vi "ToMotor2CommandSelectFunction.vi"(0 "Switch A Latched":bool=TRUE, 1 "Array":i32[][](array[numeric]), 5 "dt in sec":dbl, 7 "Potentiometer bias (-1 to +1)":dbl, 9 "Encoder 1 count":i64, 11 "Encoder 2 count":i64, 12 "Motor steps 1":i64, 13 "Motor steps 2":i64, 14 "Elapsed Time Out (S)":dbl) -> (4 "Stop":bool, 6 "Motor 1 command":i8=-1, 8 "Motor 2 command":i8=1, 10 "MS lines":bool[](array[boolean]))   [LabVIEW 2014]
panel:
  out "Integer to be added/subtracted":dbl
  out "X0":i32
  out "Y0":i32
  out "X1":i32
  out "Y1":i32
  # "Outputs"
  # "Inputs"
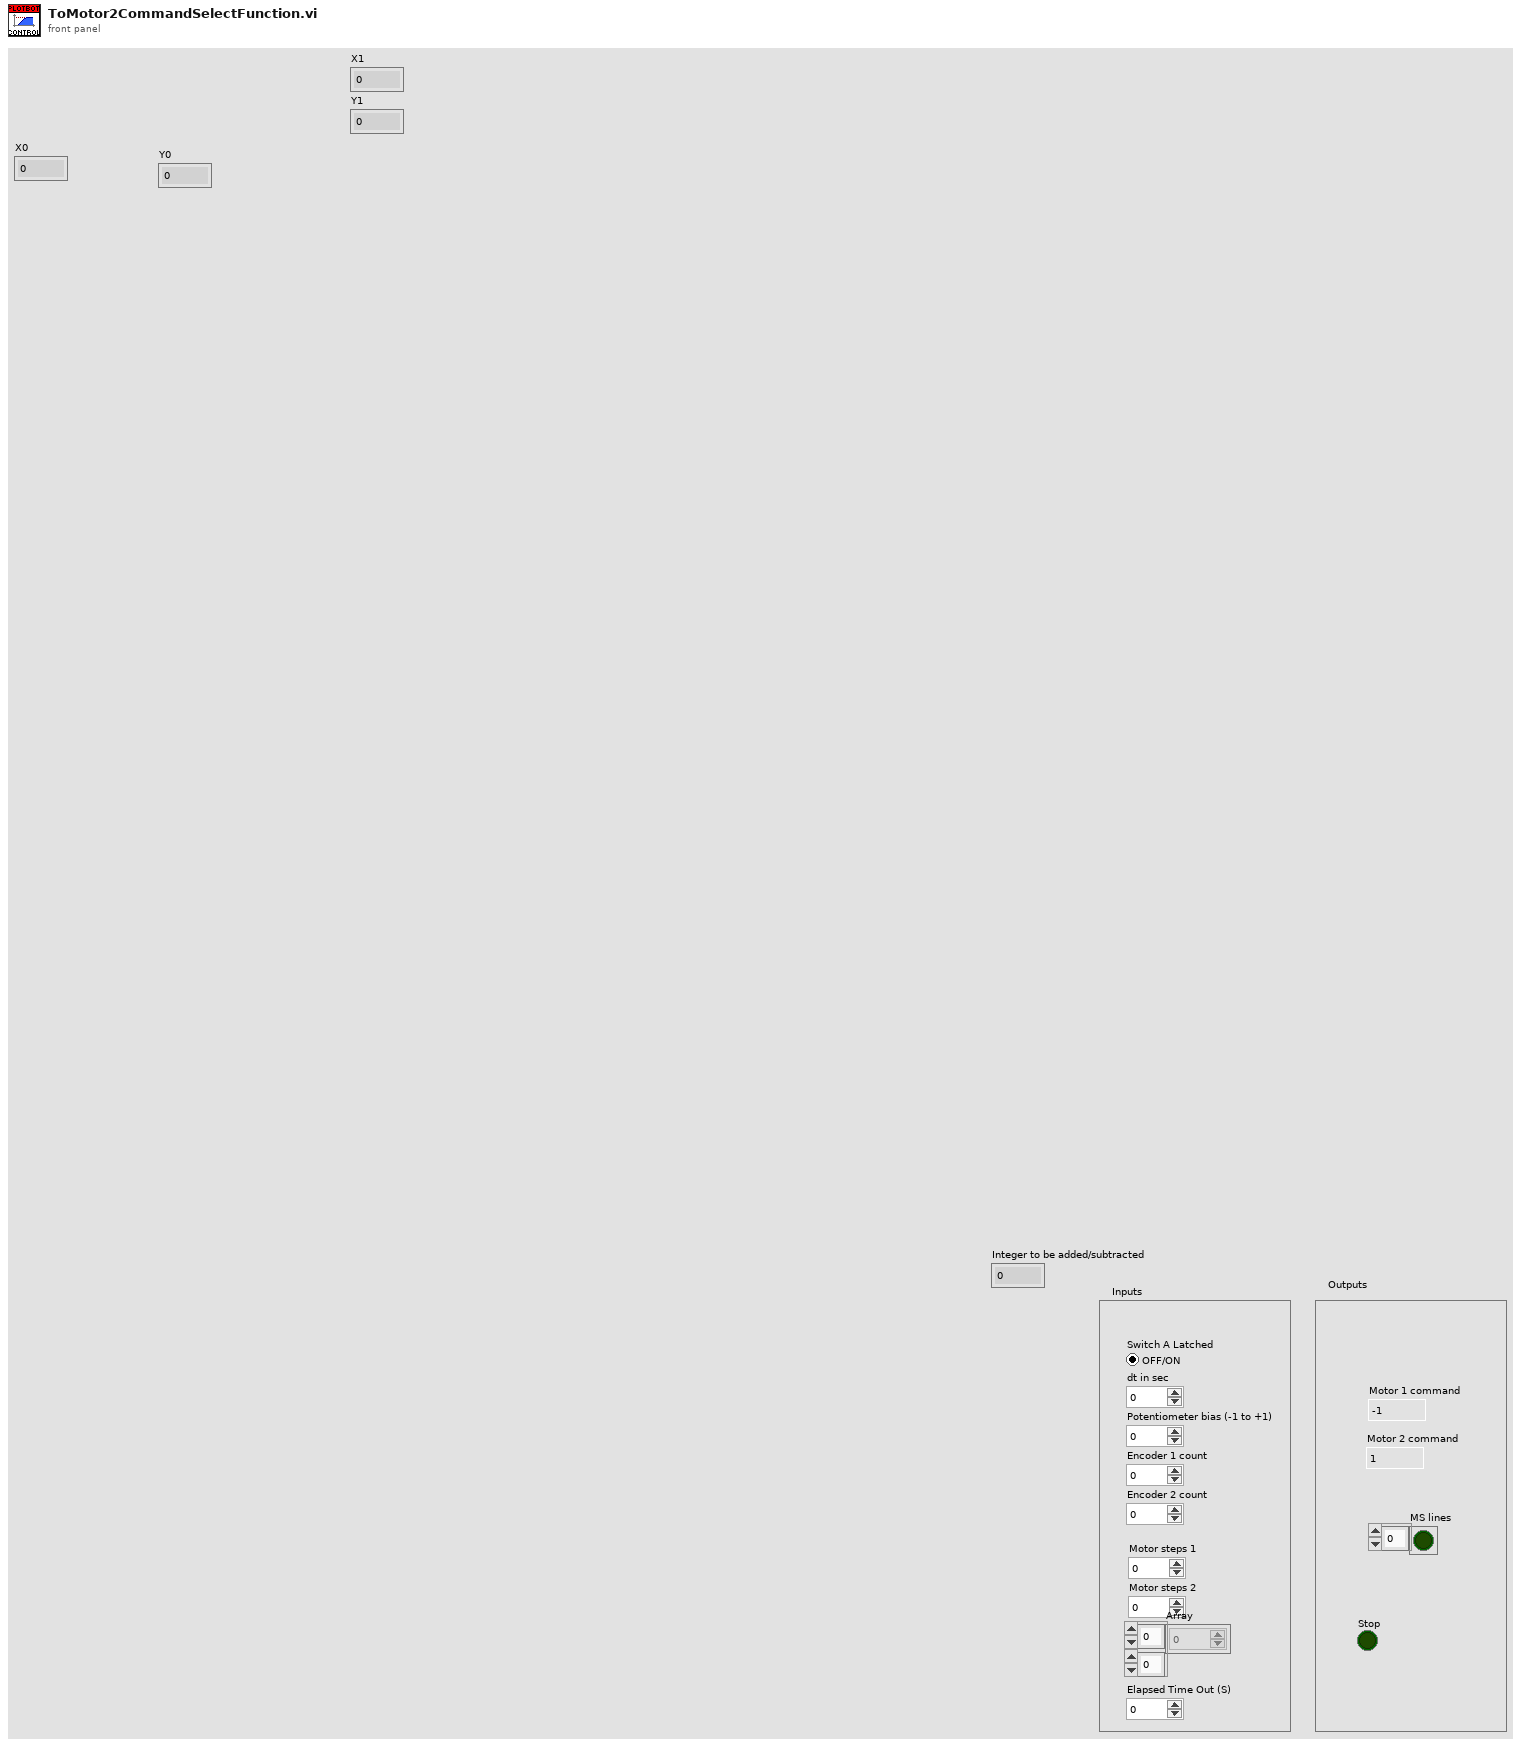
[diagram p1: front panel]
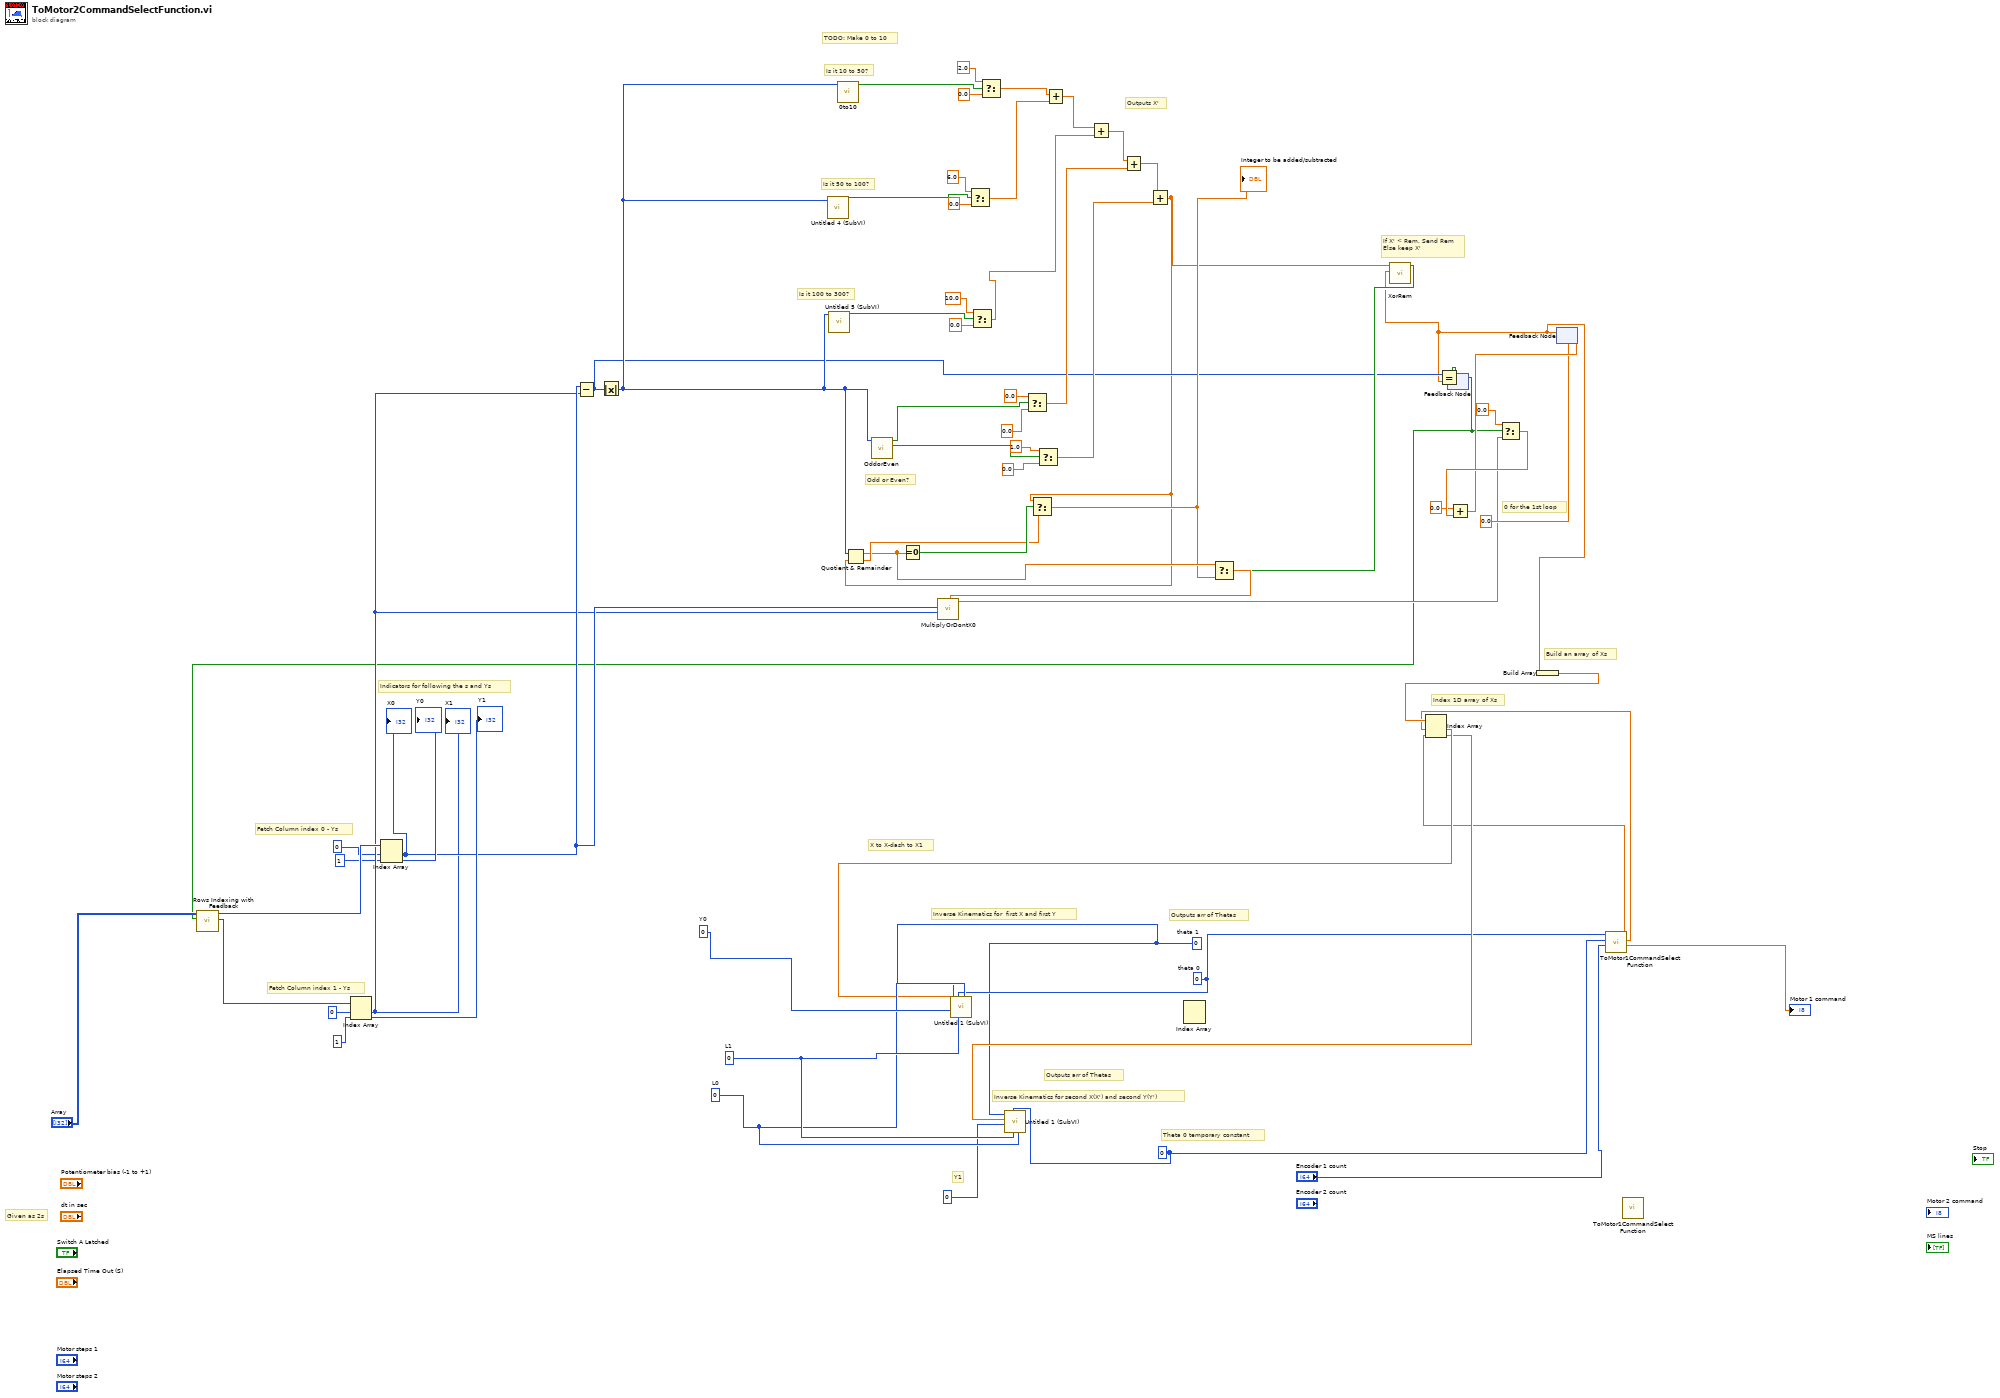
[diagram p0: block diagram]
diagram:
  w5 = 0 ("theta 0")
  w8 = 0  # theta 0
  w6 = 0  # theta 1
  w18 = 0  # L0
  w19 = 0  # L1
  w66 = 0  # Y0
  # "Theta 0 temporary constant"
  # "Y1"
  # "Fetch Column index 1 - Ys"
  # "Fetch Column index 0 - Ys"
  # "Build an array of Xs"
  # "TODO: Make 0 to 10"
  # "Outputs arr of Thetas"
  # "Outputs arr of Thetas"
  # "Inverse Kinematics for second X(X') and second Y(Y')"
  # "X to X-dash to X1"
  # "Inverse Kinematics for  first X and first Y"
  # "Index 1D array of Xs"
  # "Given as 2s"
  # "Outputs X'"
  # "If X' < Rem, Send Rem\nElse keep X'"
  # "Odd or Even?"
  # "Is it 100 to 300?"
  # "Is it 50 to 100?"
  # "Is it 10 to 50?"
  # "0 for the 1st loop"
  # "Indicators for following the s and Ys"
  n1 = Index Array() -> ()  [unwired: 3 in, 2 out]
  n2 = feedback #1() -> (w11:bool)  [unwired: 1 in]
  n3 = call "Rows Indexing with Feedback.vi"("Boolean"=w11, "Array 3"="Array") -> ("Array"=w63:i32[], "Array 2"=w64:i32[])  [unwired: 8 in]
  n4 = Index Array(array=w63, index #1=0 ("index"), index #2=1 ("index")) -> (element #1=w32:i32, element #2=→"Y1":i32)
  "X1" <- w32
  n5 = Index Array(array=w64, index #1=0 ("index"), index #2=1 ("index")) -> (element #1=w33:i32, element #2=→"Y0":i32)
  "X0" <- w33
  n6 = Subtract(x=w33, y=w32) -> (x-y=w23:i32)
  n7 = Absolute Value(x=w23) -> (abs(x)=w30:i32)
  n8 = call "Untitled 4 (SubVI).vi"("Numeric"=w30) -> ("Boolean"=w51:bool)  [unwired: 10 in]
  n9 = call "Untitled 5 (SubVI).vi"("Numeric"=w30) -> ("Boolean"=w48:bool)  [unwired: 10 in]
  n10 = call "0to10.vi"("Numeric"=w30) -> ("Boolean"=w56:bool)  [unwired: 10 in]
  n11 = call "OddorEven.vi"("Numeric"=w30) -> ("Boolean"=w46:bool, "Boolean 2"=w47:bool)  [unwired: 9 in]
  n12 = Select(t=6.0, s=w51, f=0.0) -> (s? t:f=w40:dbl)
  n13 = Select(t=10.0, s=w48, f=0.0) -> (s? t:f=w38:dbl)
  n14 = Select(t=2.0, s=w56, f=0.0) -> (s? t:f=w41:dbl)
  n15 = Select(t=0.0, s=w47, f=0.0) -> (s? t:f=w36:dbl)
  n16 = Select(t=1.0, s=w46, f=0.0) -> (s? t:f=w34:dbl)
  n17 = Add(x=w41, y=w40) -> (x+y=w39:dbl)
  n18 = Add(x=w39, y=w38) -> (x+y=w37:dbl)
  n19 = Add(x=w37, y=w36) -> (x+y=w35:dbl)
  n20 = Add(x=w35, y=w34) -> (x+y=w22:dbl)
  n21 = Quotient & Remainder(x=w30, y=w22) -> (x-y*floor(x/y)=w27:dbl, floor(x/y)=w28:dbl)
  n22 = Equal To 0?(x=w27) -> (x = 0?=w29:bool)
  n23 = Select(t=w22, s=w29, f=w28) -> (s? t:f=w26:dbl)
  "Integer to be added/subtracted" <- w26
  n24 = feedback #2(0.0) -> (w20:dbl)
  n25 = call "XorRem.vi"("Numeric 2"=w20, "Numeric"=w22) -> ("Boolean"=w24:bool)  [unwired: 9 in]
  n26 = Select(t=w27, s=w24, f=w26) -> (s? t:f=w25:dbl)
  n27 = call "MultiplyOrDontX0.vi"("Numeric 3"=w32, "Numeric 4"=w33, "Numeric in"=w25) -> ("Numeric out"=w31:dbl)  [unwired: 8 in]
  n28 = Equal?(x=w23, y=w20) -> (x = y?=w12:bool)
  n29 = feedback-in #1(w12) -> ()
  n30 = Select(t=0.0, s=w11, f=w31) -> (s? t:f=w60:dbl)
  n31 = Add(x=0.0, y=w60) -> (x+y=w59:dbl)
  n32 = Build Array(w20) -> (w17:dbl[])
  n33 = feedback-in #2(w59) -> ()
  n34 = call "ToMotor1CommandSelectFunction.vi"("Encoder 1 count"="Encoder 1 count", "theta 0"=w5, "theta 1"=w8) -> ("t"=→"Motor 1 command":dbl, "Numeric 2"=w2:dbl, "Numeric"=w1:dbl)  [unwired: 6 in]
  n35 = Index Array(array=w17, index #1=w2, index #2=w1) -> (element #1=w10:dbl, element #2=w9:dbl)
  n36 = call "Untitled 1 (SubVI).vi"("L0"=w18, "L1"=w19, "theta 0"=w8, "Y1"=w66, "X1"=w10, "theta 1"=w6) -> ()  [unwired: 6 in]
  n37 = call "Untitled 1 (SubVI).vi"("L0"=w18, "L1"=w19, "theta 0"=w5, "Y1"=0, "X1"=w9, "theta 1"=w6) -> ()  [unwired: 6 in]
  n38 = call "ToMotor1CommandSelectFunction.vi"() -> ()  [unwired: 9 in, 3 out]
